vi "Get.vi"(8 "error in (no error)":errorcluster, 11 "HW-201 in":refnum<class "HW-201.lvclass">) -> (0 "error out":errorcluster, 2 "isOnLine":bool, 3 "HW-201 out":refnum<class "HW-201.lvclass">)   [LabVIEW 2022 SP3, in "HW-201.lvlib" / "HW-201.lvclass"]
uses:
  HW-201.lvclass
  HW-201.lvclass/HW-201.ctl
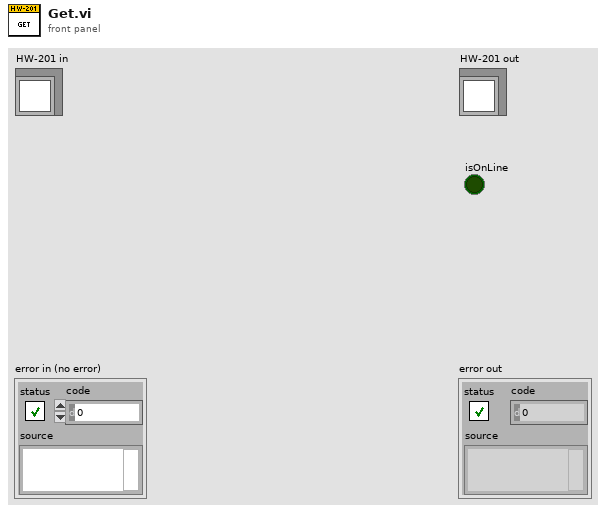
[diagram p1: front panel]
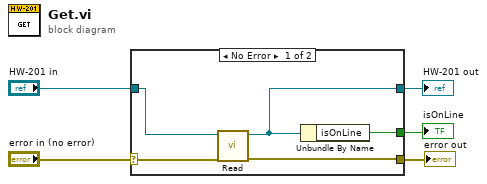
[diagram p0: block diagram]
diagram:
  n1 = case shown="No Error" "error in (no error)" {
    selector: "error in (no error)" -> [w10 w12]
    tunnel: [w8 w12] -> w4
    tunnel: [w7 w11] -> w2
    tunnel: "HW-201 in" -> [w9 w11]
    tunnel: [w6 _] -> w1
    frame No Error {
      n2 = call "Read.vi"("error in (no error)"=w10, "HW-201 in"=w9) -> ("error out"=w8:errorcluster, "HW-201 out"=w7:refnum<class "HW-201.lvclass">)  [unwired: 8 in]
      n3 = Unbundle By Name(w7) -> ("isOnLine"=w6:bool)
    }
    frame Error {
    }
  }
  "error out" <- w4
  "HW-201 out" <- w2
  "isOnLine" <- w1
